vi "proportional_power.vi"(0 "Temp":dbl, 7 "Control Parameters":T1={"Setpoint"=50.0, "Control bandwidth"=4.0, "Settle bandwidth"=1.0, "Integral time"=30.0, "Int\non"=TRUE, "Derivative time"=0.5, "Der\non"=TRUE, "Settle time"=60.0} {"Settle time" format="%.2f"; "Derivative time" format="%.2f"; "Integral time" format="%.2f"; "Settle bandwidth" format="%.2f"; "Control bandwidth" format="%.2f"; "Setpoint" format="%.2f"}) -> (4 "Normalized Power":dbl, 8 "In Range?":bool)   [LabVIEW 2016]
uses:
  typedefs/control parameters.ctl
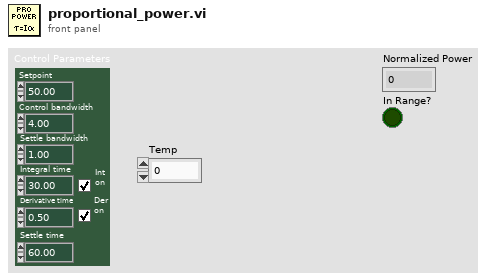
[diagram p1: front panel]
types:
  T1 = typedef "control parameters.ctl" = cluster{"Setpoint":dbl, "Control bandwidth":dbl, "Settle bandwidth":dbl, "Integral time":dbl, "Int\non":bool, "Derivative time":dbl, "Der\non":bool, "Settle time":dbl}
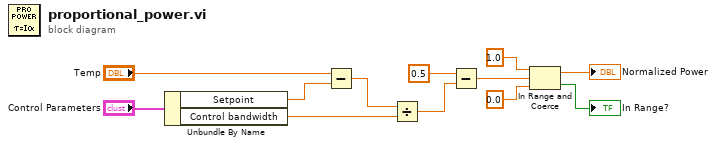
[diagram p0: block diagram]
diagram:
  n1 = Unbundle By Name("Control Parameters") -> ("Setpoint"=w10:dbl, "Control bandwidth"=w9:dbl)
  n2 = Subtract(x="Temp", y=w10) -> (x-y=w8:dbl)
  n3 = Divide(x=w8, y=w9) -> (x/y=w6:dbl)
  n4 = Subtract(x=0.5, y=w6) -> (x-y=w5:dbl)
  n5 = In Range and Coerce(upper limit=1.0, x=w5, lower limit=0.0) -> (coerced(x)=→"Normalized Power":dbl, In Range?=→"In Range?":bool)
